vi "CLD3 FGV Timer Solution 2.vi"(8 "Error In":errorcluster, 10 "Time Target (s)":dbl=4.0, 11 "Timer Mode":T1) -> (0 "Error Out":errorcluster, 2 "Has Time Elapsed":bool, 3 "Elapsed Time (s.ss)":dbl)   [LabVIEW 2019]
doc: "CLD 3 Exercise"
uses:
  CLD3 FGV Mode.ctl
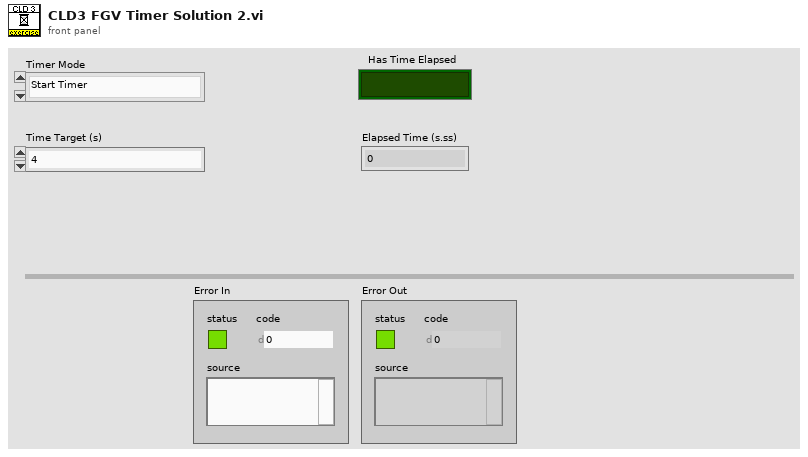
[diagram p1: front panel]
types:
  T1 = typedef "CLD3 FGV Mode.ctl" = enum16{"Start Timer", "Reset Timer", "Read Time", "Pause", "Resume"}
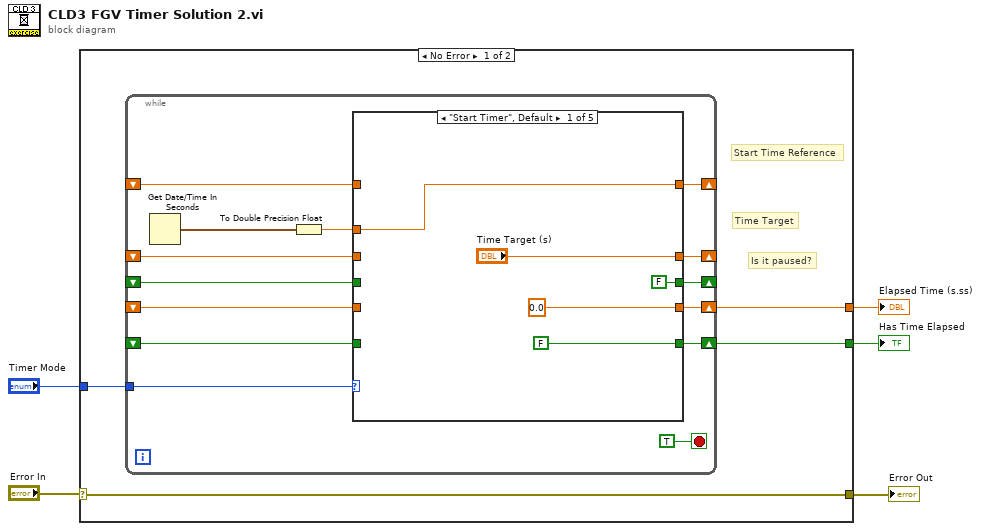
[diagram p0: block diagram]
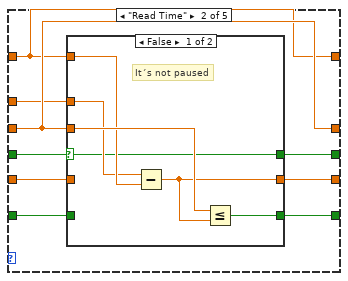
[diagram p2: hidden frame]
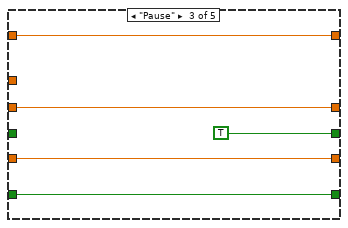
[diagram p4: hidden frame]
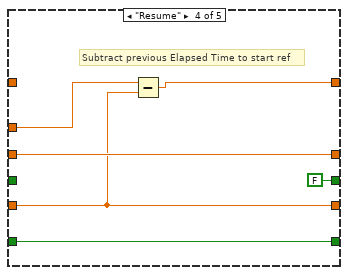
[diagram p5: hidden frame]
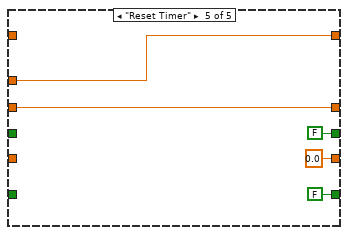
[diagram p6: hidden frame]
diagram:
  n1 = case shown="No Error" "Error In" {
    selector: "Error In" -> [w6 w63]
    tunnel: "Timer Mode" -> [w9 _]
    tunnel: [w8 _] -> w4
    tunnel: [w7 _] -> w3
    tunnel: [w6 w63] -> w1
    frame No Error {
      # "Is it paused?"
      # "Time Target"
      # "Start Time Reference"
      n2 = while {
        tunnel: w9 -> [w23]
        shift-right: [w22] -> _
        shift-left: _ -> [w18]
        shift-right: [w20] -> _
        shift-left: _ -> [w17]
        shift-right: [w19] -> w8
        shift-left: _ -> [w15]
        shift-right: [w16] -> w7
        shift-left: _ -> [w12]
        shift-right: [w11] -> _
        shift-left: _ -> [w10]
        stop <- TRUE stop-if-true
        n3 = Get Date/Time In Seconds() -> (seconds since 1Jan1904=w14:timestamp)
        n4 = To Double Precision Float(number=w14) -> (double precision float=w13:dbl)
        n5 = case shown="\"Start Timer\", Default" w23 {
          tunnel: [w25 w34 w48 w54 w62] -> w22
          tunnel: ["Time Target (s)" w37 w51 w57 w61] -> w20
          tunnel: [0.0 ("Time Target (s)") w36 w50 w55 0.0 ("Time Target (s)")] -> w19
          tunnel: w18 -> [_ w34 w48 _ _]
          tunnel: w17 -> [_ w37 w51 w57 w61]
          tunnel: [FALSE w35 w49 w56 FALSE] -> w16
          tunnel: w15 -> [_ w30 w50 w55 _]
          tunnel: w13 -> [w25 w33 _ w53 w62]
          tunnel: w12 -> [_ w31 w49 w56 _]
          tunnel: [FALSE w29 TRUE FALSE FALSE] -> w11
          tunnel: w10 -> [_ w32 _ _ _]
          frame "Start Timer", Default {
          }
          frame "Read Time" {
            n6 = case shown="False" w32 {
              selector: w32 -> [w38 w44]
              tunnel: w37 -> [w43 _]
              tunnel: [w42 w45] -> w36
              tunnel: [w41 w46] -> w35
              tunnel: w34 -> [w40 _]
              tunnel: w33 -> [w39 _]
              tunnel: w31 -> [_ w46]
              tunnel: w30 -> [_ w45]
              tunnel: [w38 w44] -> w29
              frame False {
                # "It´s not paused"
                n7 = Subtract(x=w39, y=w40) -> (x-y=w42:dbl)
                n8 = Less Or Equal?(x=w43, y=w42) -> (x <= y?=w41:bool)
              }
              frame True {
              }
            }
          }
          frame "Pause" {
          }
          frame "Resume" {
            # "Subtract previous Elapsed Time to start ref"
            n9 = Subtract(x=w53, y=w55) -> (x-y=w54:dbl)
          }
          frame "Reset Timer" {
          }
        }
      }
    }
    frame Error {
    }
  }
  "Error Out" <- w1
  "Elapsed Time (s.ss)" <- w4
  "Has Time Elapsed" <- w3
